vi "LlenarColumnadeTabla.vi"(9 "Data":string[](array[string]), 10 "Col. Number":i32, 11 "Tabla in":string[][](array[string])) -> (3 "Tabla out":string[][](array[string]))   [LabVIEW 2019, in "Prueba031.lvclass"]
uses:
  Prueba031.lvclass
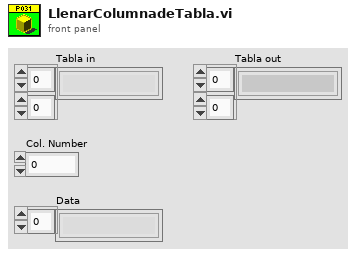
[diagram p1: front panel]
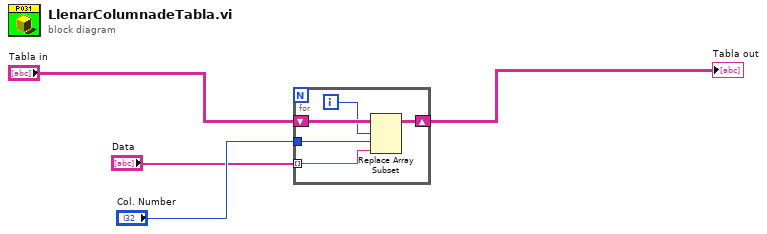
[diagram p0: block diagram]
diagram:
  n1 = for {
    tunnel: "Data" -> [w6] mode=indexing
    tunnel: "Col. Number" -> [w7]
    shift-right: [w5] -> w2
    shift-left: "Tabla in" -> [w9]
    i -> [w8]
    n2 = Replace Array Subset(array=w9, new element=w6, index (row)=w8, index (col)=w7) -> (w5:string[][])
  }
  "Tabla out" <- w2
